vi "FlatToRichcif_channelcore_FIFOInstance.vi"(5 "OutputClusterType":T1, 11 "InputCluster":T2) -> (3 "OutputCluster":T1)   [LabVIEW 2021, in "CIF_Launcher_client.lvlib"]
uses:
  CIF_Launcher_client.lvlib
  cif_channelcore_FIFOInstance_Flat.ctl
  cif_channelcore_FIFOInstance.ctl
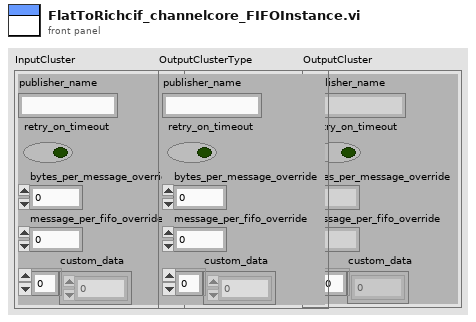
[diagram p1: front panel]
types:
  T1 = typedef "CIF_Launcher_client.lvlib/cif_channelcore_FIFOInstance.ctl" = cluster{"publisher_name":string, "retry_on_timeout":bool, "bytes_per_message_override":u32, "message_per_fifo_override":u32, "custom_data":u8[]}
  T2 = typedef "CIF_Launcher_client.lvlib/cif_channelcore_FIFOInstance_Flat.ctl" = cluster{"publisher_name":string, "retry_on_timeout":bool, "bytes_per_message_override":u32, "message_per_fifo_override":u32, "custom_data":u8[]}
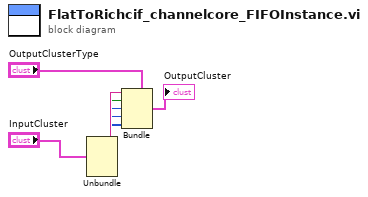
[diagram p0: block diagram]
diagram:
  n1 = Unbundle "Unbundle"("InputCluster") -> ("publisher_name"=w5:string, "retry_on_timeout"=w4:bool, "bytes_per_message_override"=w3:u32, "message_per_fifo_override"=w2:u32, "custom_data"=w1:u8[])
  n2 = Bundle "Bundle"(cluster="OutputClusterType", "publisher_name"=w5, "retry_on_timeout"=w4, "bytes_per_message_override"=w3, "message_per_fifo_override"=w2, "custom_data"=w1) -> (→"OutputCluster":T1)
